vi "Quick Start - Workspaces.vi"   [LabVIEW 2020]
uses:
  b8c625b9-7f41-4907-b61e-90a3f4e11cd5.vi
  Nominal Client/Nominal Client.lvclass
  d5fec867-f3f3-4b59-a900-6f7a14bb6c1f.vi
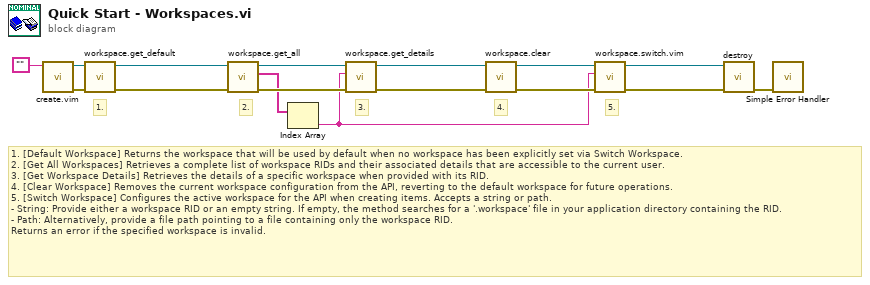
[diagram p0: block diagram]
diagram:
  # "5."
  # "4."
  # "3."
  # "2."
  # "1."
  # "1. [Default Workspace] Returns the workspace that will be used by default when no workspace has been explicitly set via Switch Workspace.\n2. [Get All Workspaces] Retrieves a complete list of workspace RIDs and their associated details that are accessible to the current user.\n3. [Get Workspace Details] Retrieves the details of a specific workspace when provided with its RID.\n4. [Clear Workspace] Removes the current workspace configuration from the API, reverting to the default workspace for future operations.\n5. [Switch Workspace] Configures the active workspace for the API when creating items. Accepts a string or path.\n- String: Provide either a workspace RID or an empty string. If empty, the method searches for a '.workspace' file in your application directory containing the RID.\n- Path: Alternatively, provide a file path pointing to a file containing only the workspace RID.\nReturns an error if the specified workspace is invalid."
  n1 = call "create.vim"("API Token (string or path)"="") -> ("error out"=w14:errorcluster, "Nominal Client"=w15:refnum<class "Nominal Client.lvclass">)  [unwired: 9 in]
  n2 = call "workspace.get_default.vi"("error in"=w14, "Nominal Client in"=w15) -> ("error out"=w12:errorcluster, "Nominal Client out"=w13:refnum<class "Nominal Client.lvclass">)  [unwired: 6 in, 2 out]
  n3 = call "workspace.get_all.vi"("error in"=w12, "Nominal Client in"=w13) -> ("error out"=w10:errorcluster, "Workspace RIDs"=w3:string[], "Nominal Client out"=w11:refnum<class "Nominal Client.lvclass">)  [unwired: 5 in, 2 out]
  n4 = Index Array(array=w3) -> (element=w2:string)  [unwired: 1 in]
  n5 = call "workspace.get_details.vi"("error in"=w10, "Workspace RID"=w2, "Nominal Client in"=w11) -> ("error out"=w8:errorcluster, "Nominal Client out"=w9:refnum<class "Nominal Client.lvclass">)  [unwired: 5 in, 2 out]
  n6 = call "workspace.clear.vi"("error in"=w8, "Nominal Client in"=w9) -> ("error out"=w6:errorcluster, "Nominal Client out"=w7:refnum<class "Nominal Client.lvclass">)  [unwired: 8 in]
  n7 = call "workspace.switch.vim"("error in"=w6, "Workspace RID (string or path)"=w2, "Nominal Client in"=w7) -> ("error out"=w4:errorcluster, "Nominal Client out"=w5:refnum<class "Nominal Client.lvclass">)  [unwired: 7 in]
  n8 = call "destroy.vi"("error in"=w4, "Nominal Client"=w5) -> ("error out"=w1:errorcluster)  [unwired: 9 in]
  n9 = call <vilib>:"Simple Error Handler.vi"("error in (no error)"=w1) -> ()  [unwired: 4 in, 5 out]
